vi "tc_selection_new.vi"(9 "Numeric 2":i32=5, 10 "Coords":T1, 11 "Position":T2) -> (3 "Numeric":i32)   [LabVIEW 2017]
uses:
  <vilib>/Utility/miscctls.llb/LVPositionTypeDef.ctl
  <vilib>/Utility/miscctls.llb/LVPoint32TypeDef.ctl
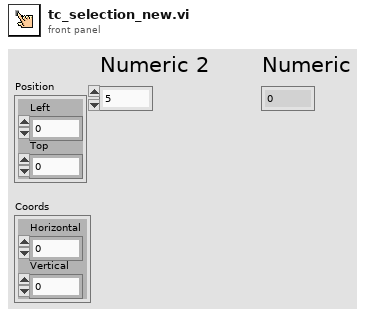
[diagram p1: front panel]
types:
  T1 = typedef "LVPoint32TypeDef.ctl" = cluster{"Horizontal":i32, "Vertical":i32}
  T2 = typedef "LVPositionTypeDef.ctl" = cluster{"Left":i32, "Top":i32}
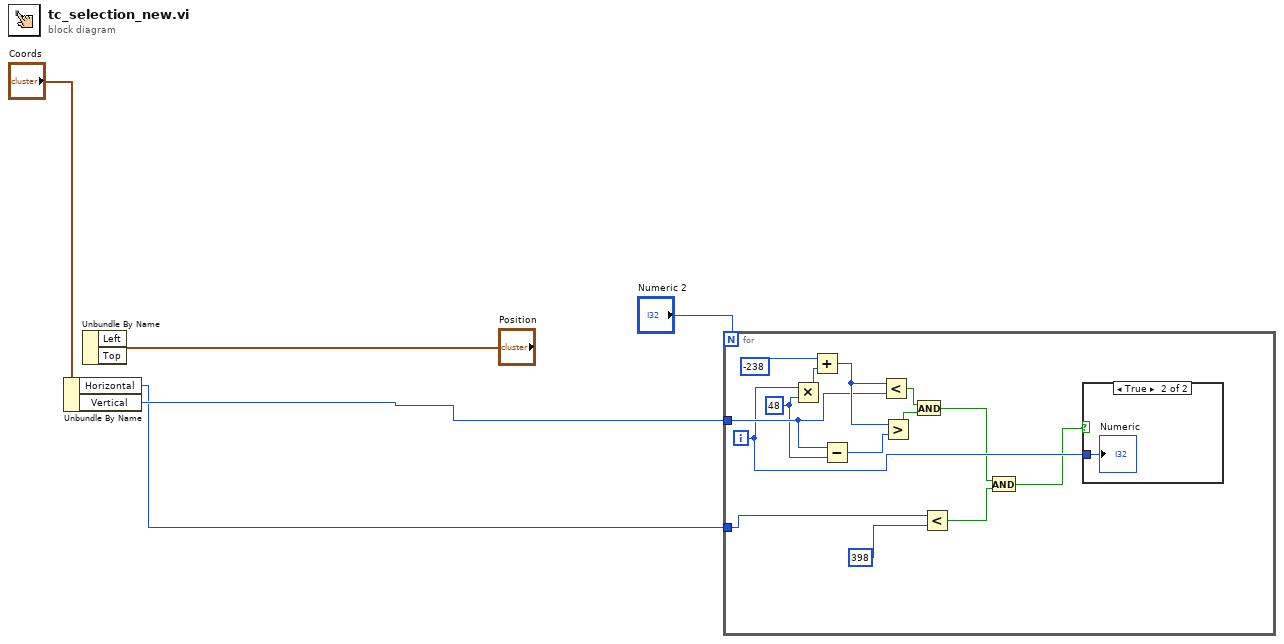
[diagram p0: block diagram]
diagram:
  n1 = Unbundle By Name("Coords") -> ("Horizontal"=w1:i32, "Vertical"=w2:i32)
  n2 = Unbundle By Name("Position") -> ()  [unwired: 2 out]
  n3 = for {
    N: "Numeric 2" -> [_]
    tunnel: w2 -> [w15]
    tunnel: w1 -> [w7]
    i -> [w11]
    w14 = 48
    n4 = Multiply(x=w11, y=w14) -> (x*y=w19:i32)
    n5 = Add(x=-238, y=w19) -> (x+y=w17:i32)
    n6 = Subtract(x=w15, y=w14) -> (x-y=w16:i32)
    n7 = Less?(x=w17, y=w15) -> (x < y?=w12:bool)
    n8 = Greater?(x=w17, y=w16) -> (0:w13:bool)
    n9 = And(x=w12, y=w13) -> (x .and. y?=w9:bool)
    n10 = Less?(x=w7, y=398) -> (x < y?=w6:bool)
    n11 = And(x=w9, y=w6) -> (x .and. y?=w10:bool)
    n12 = case shown="True" w10 {
      tunnel: w11 -> [_ w20]
      frame False {
      }
      frame True {
        "Numeric" <- w20
      }
    }
  }
